vi "Not A DSF Configuration Refnum.vi"(1 "Configuration Session":refnum<class "Configuration.lvclass">) -> (0 "not a dsf refnum":bool)   [LabVIEW 2017, in "DSF Core.lvlib" / "Configuration.lvclass"]
doc: "Determines whether a configuration data dsf refnum is valid."
uses:
  Configuration.lvclass
  Configuration.lvclass/Configuration.ctl
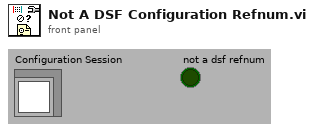
[diagram p1: front panel]
types:
  T1 = typedef "DSF Core.lvlib/Configuration.lvclass/DSF Config Data Ref.ctl" = refnum<data-value>
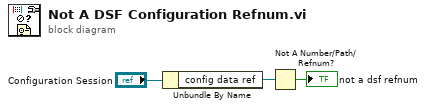
[diagram p0: block diagram]
diagram:
  n1 = Unbundle By Name("Configuration Session") -> ("config data ref"=w1:T1)
  n2 = Not A Number/Path/Refnum?(number/path/refnum=w1) -> (NaN/Path/Refnum?=→"not a dsf refnum":bool)
